vi "Close.vi"(8 "error in (no error)":errorcluster, 10 "Internal?":bool, 11 "Julabo Fp-50 Settings":T1={"VISA resource name"="", "Simulated?"=FALSE, "Pump Power"=2} {"Pump Power" min=0 max=8 step=1}) -> (0 "error out":errorcluster, 3 "Julabo FP-50 Settings":T1={"VISA resource name"="", "Simulated?"=FALSE, "Pump Power"=2} {"Pump Power" min=0 max=8 step=1})   [LabVIEW 2018, in "Julabo Type FP-50 TCU.lvlib"]
uses:
  Julabo Type FP-50 TCU.lvlib
  Julabo FP-50 Settings.ctl
  Third Party Drivers/Julabo Type 1/JULABO DeviceDriver/JULABO DeviceDriver.lvlib
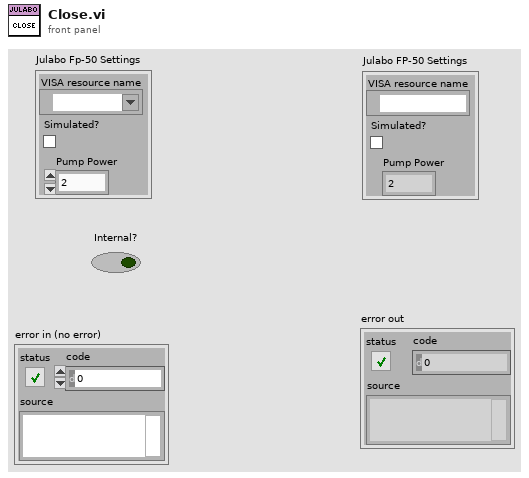
[diagram p1: front panel]
types:
  T1 = typedef "Julabo Type FP-50 TCU.lvlib/Julabo FP-50 Settings.ctl" = cluster{"VISA resource name":refnum<visa-resource-name>, "Simulated?":bool, "Pump Power":i32}
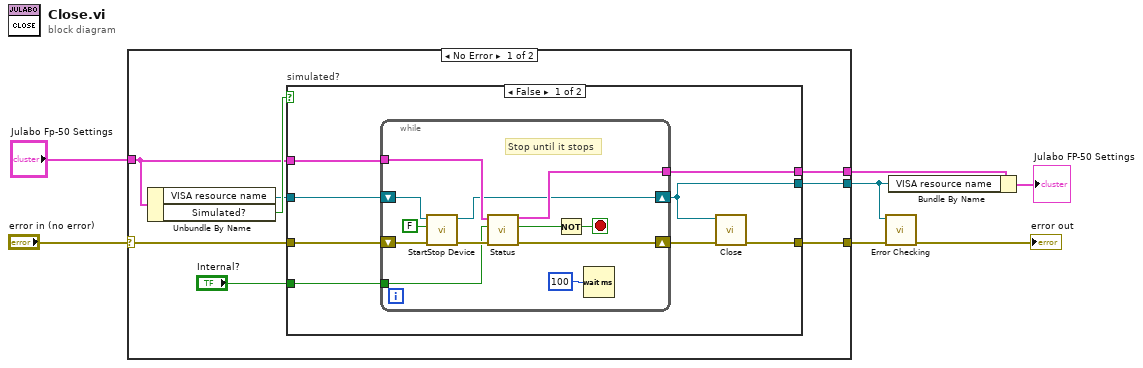
[diagram p0: block diagram]
diagram:
  n1 = case shown="No Error" "error in (no error)" {
    selector: "error in (no error)" -> [w13 w41]
    tunnel: [w14 w41] -> w6
    tunnel: "Julabo Fp-50 Settings" -> [w10 w39]
    tunnel: [w11 w40] -> w4
    tunnel: [w9 w39] -> w3
    frame No Error {
      n2 = Unbundle By Name(w10) -> ("VISA resource name"=w12:refnum<visa-resource-name>, "Simulated?"=w15:bool)
      n3 = case "simulated?" shown="False" w15 {
        tunnel: [w18 w38] -> w14
        tunnel: w12 -> [w22 w37]
        tunnel: w13 -> [w23 w38]
        tunnel: [w17 w37] -> w11
        tunnel: w10 -> [w21 w36]
        tunnel: [w20 w36] -> w9
        tunnel: "Internal?" -> [w16 _]
        frame False {
          n4 = while {
            shift-right: [w35] -> w19
            shift-left: w23 -> [w27]
            shift-right: [w25] -> w17
            shift-left: w22 -> [w28]
            tunnel: w21 -> [w31]
            tunnel: [w32] -> w20
            tunnel: w16 -> [w24]
            stop <- w34 stop-if-true
            # "Stop until it stops"
            n5 = call "StartStop Device.vi"("error in (no error)"=w27, "Start/Stop (f:Stop)"=FALSE, "VISA resource name"=w28) -> ("error out"=w26:errorcluster, "VISA resource name out"=w25:refnum<visa-resource-name>)  [unwired: 7 in]
            n6 = call "Status.vi"("error in (no error)"=w26, "Internal?"=w24, "Julabo FP-50 Settings"=w31) -> ("error out"=w35:errorcluster, "Running"=w33:bool, "Julabo FP-50 Settings"=w32:T1)  [unwired: 3 in, 3 out]
            n7 = Not(x=w33) -> (.not. x?=w34:bool)
            n8 = Wait (ms)(milliseconds to wait=u32 100) -> ()  [unwired: 1 out]
          }
          n9 = call "Close.vi"("error in (no error)"=w19, "VISA resource name"=w17) -> ("error out"=w18:errorcluster)  [unwired: 9 in]
        }
        frame True {
        }
      }
    }
    frame Error {
      n10 = Unbundle By Name(w39) -> ("VISA resource name"=w40:refnum<visa-resource-name>)
    }
  }
  n11 = call "Error Checking.vi"("error in (no error)"=w6, "VISA resource name"=w4) -> ("error out"=→"error out":errorcluster)  [unwired: 7 in, 2 out]
  n12 = Bundle By Name(cluster=w3, "VISA resource name"=w4) -> (→"Julabo FP-50 Settings":T1)
